vi "ARC_Dynamic Call_Single.vi"(5 "command queue name":string, 6 "time out(5s)":dbl=5.0, 7 "open front panel? (T)":bool=TRUE, 8 "error in (no error)":errorcluster, 9 "parameter else":variant, 10 "control name":string, 11 "vi path":path) -> (0 "error out":errorcluster, 1 "time out":bool, 2 "call failed":bool)   [LabVIEW 2016]
uses:
  Queue Management/ARC_Queue Valid.vi
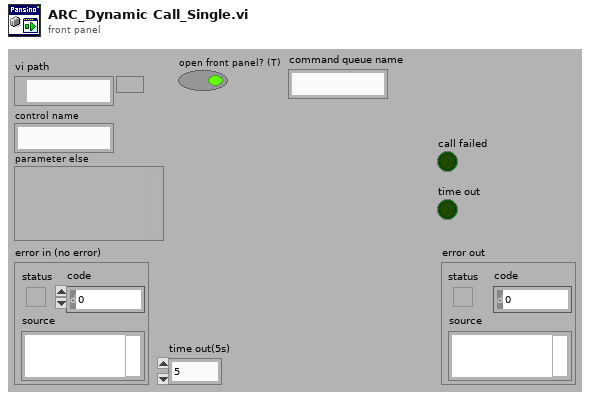
[diagram p1: front panel]
types:
  T1 = enum32{"Bad", "Idle", "Run top level", "Running"}
  T2 = enum32{"Invalid", "Standard", "Closed", "Hidden", "Minimized", "Maximized"}
  T3 = cluster{"command queue name":string, "parameter else":variant}
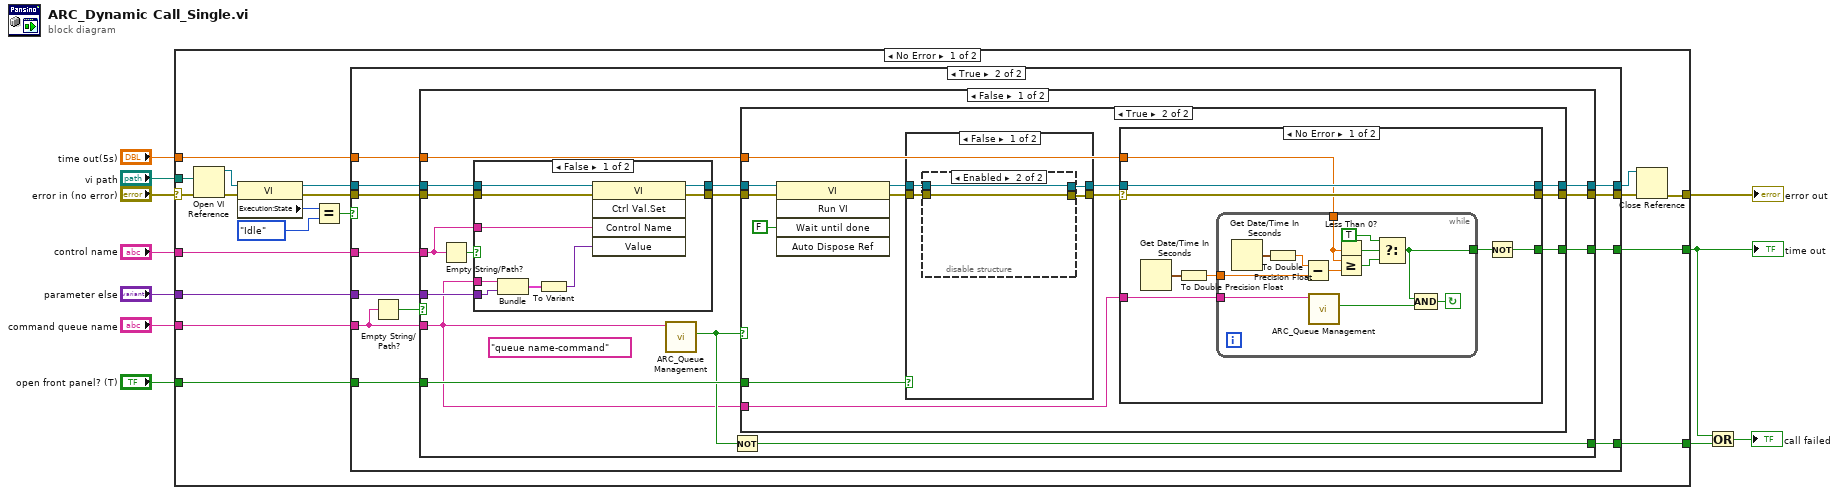
[diagram p0: block diagram]
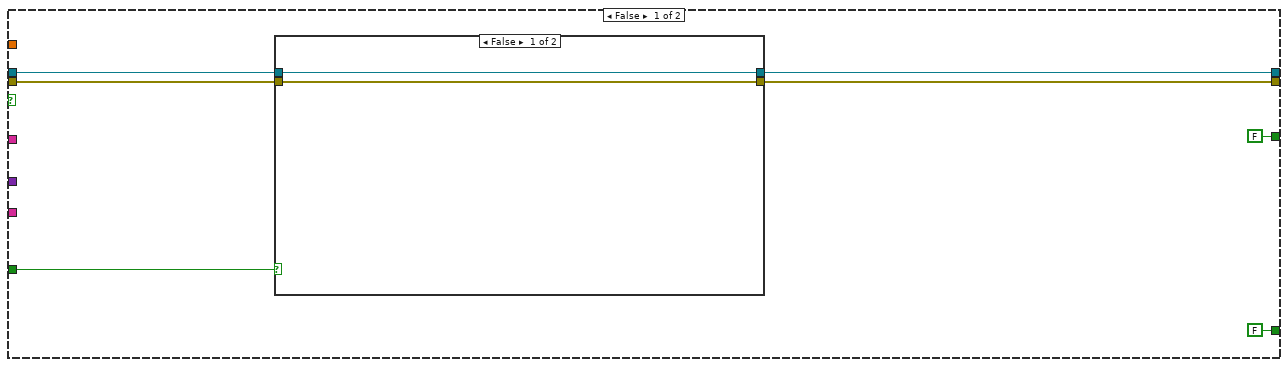
[diagram p2: hidden frame]
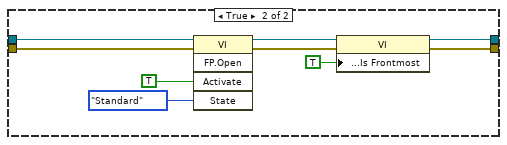
[diagram p3: hidden frame]
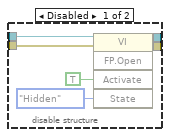
[diagram p6: hidden frame]
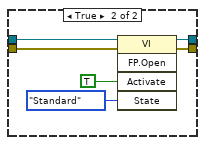
[diagram p7: hidden frame]
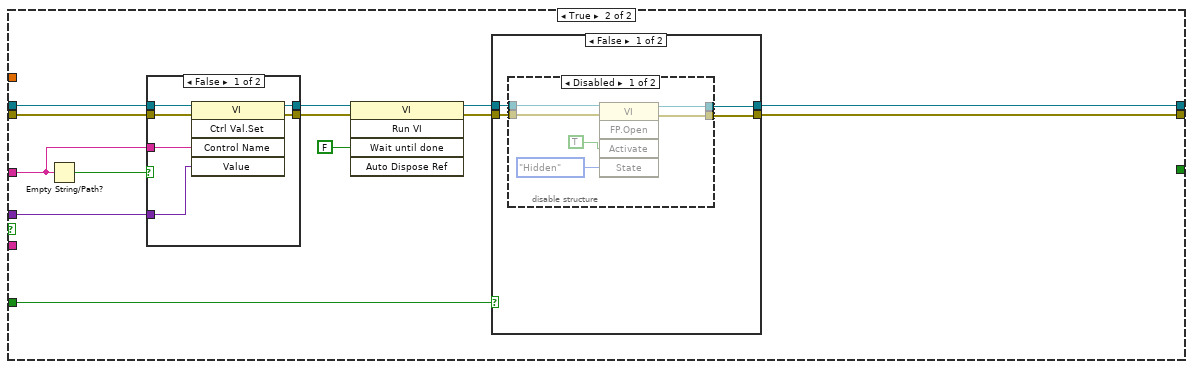
[diagram p9: hidden frame]
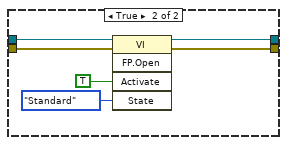
[diagram p12: hidden frame]
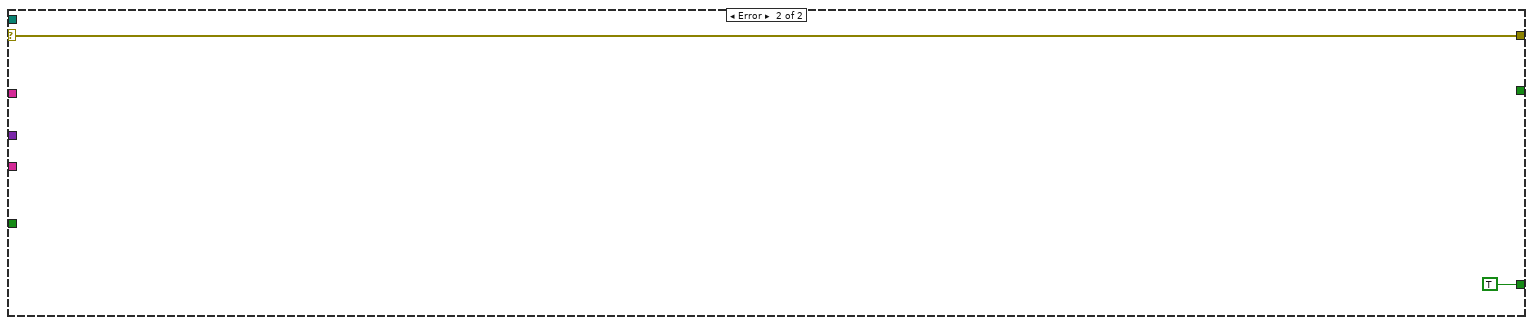
[diagram p13: hidden frame]
diagram:
  n1 = case shown="No Error" "error in (no error)" {
    selector: "error in (no error)" -> [w23 w182]
    tunnel: [w14 w182] -> w10
    tunnel: "vi path" -> [w22 _]
    tunnel: "open front panel? (T)" -> [w21 _]
    tunnel: "control name" -> [w20 _]
    tunnel: "command queue name" -> [w19 _]
    tunnel: "parameter else" -> [w18 _]
    tunnel: "time out(5s)" -> [w17 _]
    tunnel: [w16 TRUE] -> w3
    tunnel: [w15 _] -> w2
    frame No Error {
      n2 = Open VI Reference(vi path=w22, error in (no error)=w23) -> (vi reference=w25:refnum<vi>, error out=w27:errorcluster)  [unwired: 4 in]
      n3 = property class="VI"(reference=w25, error in=w27) -> (reference out=w28:refnum<vi>, error out=w26:errorcluster, "Execution:State"=w30:T1)
      n4 = Equal?(x=w30, y=T1."Idle") -> (x = y?=w24:bool)
      n5 = case shown="True" w24 {
        tunnel: [w34 w60] -> w12
        tunnel: [w35 w59] -> w13
        tunnel: w28 -> [w37 w57]
        tunnel: w26 -> [w36 w56]
        tunnel: w21 -> [w33 w58]
        tunnel: w20 -> [_ w55]
        tunnel: w19 -> [_ w54]
        tunnel: w18 -> [_ w53]
        tunnel: w17 -> [_ w51]
        tunnel: [FALSE w50] -> w16
        tunnel: [FALSE w49] -> w15
        frame False {
          n6 = case shown="False" w33 {
            tunnel: w37 -> [w39 w44]
            tunnel: w36 -> [w38 w42]
            tunnel: [w38 w48] -> w35
            tunnel: [w39 w47] -> w34
            frame False {
            }
            frame True {
              n7 = invoke class="VI" method="FP.Open"(reference=w44, error in=w42, "Activate"=TRUE ("激活？"), "State"=T2."Standard" ("状态")) -> (reference out=w43:refnum<vi>, error out=w41:errorcluster)  [unwired: 1 in, 3 out]
              n8 = property class="VI"(reference=w43, error in=w41, "Front Panel Window:Is Frontmost"=TRUE) -> (reference out=w47:refnum<vi>, error out=w48:errorcluster)
            }
          }
        }
        frame True {
          n9 = Empty String/Path?(string/path=w54) -> (empty?=w52:bool)
          n10 = case shown="False" w52 {
            tunnel: [w75 w154] -> w60
            tunnel: [w74 w153] -> w59
            tunnel: w58 -> [w73 w152]
            tunnel: w57 -> [w72 w151]
            tunnel: w56 -> [w71 w150]
            tunnel: w55 -> [w70 w149]
            tunnel: w54 -> [w63 _]
            tunnel: w53 -> [w64 w142]
            tunnel: w51 -> [w68 _]
            tunnel: [w66 _] -> w50
            tunnel: [w65 _] -> w49
            frame False {
              (unwired) "queue name-command" ("控件名")
              n11 = Empty String/Path?(string/path=w70) -> (empty?=w69:bool)
              n12 = case shown="False" w69 {
                tunnel: w72 -> [w139 w141]
                tunnel: [w138 w141] -> w62
                tunnel: [w137 w140] -> w61
                tunnel: w71 -> [w136 w140]
                tunnel: w70 -> [w135 _]
                tunnel: w64 -> [w133 _]
                tunnel: w63 -> [w134 _]
                frame False {
                  n13 = Bundle("command queue name"=w134, "parameter else"=w133) -> (w132:T3)  [unwired: 1 in]
                  n14 = To Variant(anything=w132) -> (Variant=w131:variant)
                  n15 = invoke class="VI" method="Ctrl Val.Set"(reference=w139, error in=w136, "Control Name"=w135, "Value"=w131) -> (reference out=w138:refnum<vi>, error out=w137:errorcluster)  [unwired: 1 in, 3 out]
                }
                frame True {
                }
              }
              n16 = call-poly "ARC_Queue Management.vi"("Queue Name(unamed)"=w63) -> ("Not Exist?"=w67:bool)  [unwired: 8 in, 2 out]
              n17 = Not(x=w67) -> (.not. x?=w66:bool)
              n18 = case shown="True" w67 {
                tunnel: [w77 w82] -> w75
                tunnel: [w76 w81] -> w74
                tunnel: w73 -> [_ w90]
                tunnel: w62 -> [w77 w87]
                tunnel: w61 -> [w76 w86]
                tunnel: w63 -> [_ w79]
                tunnel: w68 -> [_ w80]
                tunnel: [_ w78] -> w65
                frame False {
                }
                frame True {
                  n19 = invoke class="VI" method="Run VI"(reference=w87, error in=w86, "Wait until done"=FALSE) -> (reference out=w88:refnum<vi>, error out=w89:errorcluster)  [unwired: 2 in, 3 out]
                  n20 = case shown="False" w90 {
                    tunnel: w89 -> [w114 w126]
                    tunnel: w88 -> [w116 w128]
                    tunnel: [w115 w127] -> w83
                    tunnel: [w113 w125] -> w84
                    frame False {
                      n21 = disable-structure shown="Enabled" {
                        disable-tunnel: w116 -> [w120 w124]
                        disable-tunnel: [w119 w124] -> w115
                        disable-tunnel: w114 -> [w118 w123]
                        disable-tunnel: [w117 w123] -> w113
                        frame Disabled {
                          n22 = invoke class="VI" method="FP.Open"(reference=w120, error in=w118, "Activate"=TRUE ("激活？"), "State"=T2."Hidden" ("状态")) -> (reference out=w119:refnum<vi>, error out=w117:errorcluster)  [unwired: 1 in, 3 out]
                        }
                        frame Enabled {
                        }
                      }
                    }
                    frame True {
                      n23 = invoke class="VI" method="FP.Open"(reference=w128, error in=w126, "Activate"=TRUE ("激活？"), "State"=T2."Standard" ("状态")) -> (reference out=w127:refnum<vi>, error out=w125:errorcluster)  [unwired: 1 in, 3 out]
                    }
                  }
                  n24 = case shown="No Error" w84 {
                    selector: w84 -> [w97 w111]
                    tunnel: w83 -> [w98 w112]
                    tunnel: [w98 w112] -> w82
                    tunnel: [w97 w111] -> w81
                    tunnel: w79 -> [w94 _]
                    tunnel: w80 -> [w93 _]
                    tunnel: [w91 _] -> w78
                    frame No Error {
                      n25 = Get Date/Time In Seconds() -> (seconds since 1Jan1904=w95:timestamp)
                      n26 = To Double Precision Float(number=w95) -> (double precision float=w96:dbl)
                      n27 = while {
                        tunnel: w96 -> [w108]
                        tunnel: w94 -> [w103]
                        tunnel: w93 -> [w102]
                        tunnel: [w99] -> w92
                        stop <- w105 continue-if-true
                        n28 = Get Date/Time In Seconds() -> (seconds since 1Jan1904=w109:timestamp)
                        n29 = To Double Precision Float(number=w109) -> (double precision float=w110:dbl)
                        n30 = Subtract(x=w110, y=w108) -> (x-y=w107:dbl)
                        n31 = call-poly "ARC_Queue Management.vi"("Queue Name(unamed)"=w103) -> ("Not Exist?"=w106:bool)  [unwired: 8 in, 2 out]
                        n32 = Less Than 0?(x=w102) -> (x < 0?=w101:bool)
                        n33 = Greater Or Equal?(x=w102, y=w107) -> (x >= y?=w104:bool)
                        n34 = Select(t=TRUE, s=w101, f=w104) -> (s? t:f=w99:bool)
                        n35 = Compound Arithmetic op=AND(w99, w106) -> (w105:bool)
                      }
                      n36 = Not(x=w92) -> (.not. x?=w91:bool)
                    }
                    frame Error {
                    }
                  }
                }
              }
            }
            frame True {
              n37 = Empty String/Path?(string/path=w149) -> (empty?=w143:bool)
              n38 = case shown="False" w143 {
                tunnel: w151 -> [w160 w162]
                tunnel: [w159 w162] -> w146
                tunnel: [w158 w161] -> w145
                tunnel: w150 -> [w157 w161]
                tunnel: w149 -> [w156 _]
                tunnel: w142 -> [w155 _]
                frame False {
                  n39 = invoke class="VI" method="Ctrl Val.Set"(reference=w160, error in=w157, "Control Name"=w156, "Value"=w155) -> (reference out=w159:refnum<vi>, error out=w158:errorcluster)  [unwired: 1 in, 3 out]
                }
                frame True {
                }
              }
              n40 = invoke class="VI" method="Run VI"(reference=w146, error in=w145, "Wait until done"=FALSE) -> (reference out=w147:refnum<vi>, error out=w148:errorcluster)  [unwired: 2 in, 3 out]
              n41 = case shown="False" w152 {
                tunnel: w148 -> [w164 w176]
                tunnel: w147 -> [w166 w178]
                tunnel: [w165 w177] -> w154
                tunnel: [w163 w175] -> w153
                frame False {
                  n42 = disable-structure shown="Disabled" {
                    disable-tunnel: w166 -> [w170 w174]
                    disable-tunnel: [w169 w174] -> w165
                    disable-tunnel: w164 -> [w168 w173]
                    disable-tunnel: [w167 w173] -> w163
                    frame Disabled {
                      n43 = invoke class="VI" method="FP.Open"(reference=w170, error in=w168, "Activate"=TRUE ("激活？"), "State"=T2."Hidden" ("状态")) -> (reference out=w169:refnum<vi>, error out=w167:errorcluster)  [unwired: 1 in, 3 out]
                    }
                    frame Enabled {
                    }
                  }
                }
                frame True {
                  n44 = invoke class="VI" method="FP.Open"(reference=w178, error in=w176, "Activate"=TRUE ("激活？"), "State"=T2."Standard" ("状态")) -> (reference out=w177:refnum<vi>, error out=w175:errorcluster)  [unwired: 1 in, 3 out]
                }
              }
            }
          }
        }
      }
      n45 = Close Reference(reference=w12, error in (no error)=w13) -> (error out=w14:errorcluster)
    }
    frame Error {
    }
  }
  "error out" <- w10
  "time out" <- w2
  n46 = Or(x=w2, y=w3) -> (x .or. y?=→"call failed":bool)
